vi "Transmit ACK.vi"(8 "error in (no error)":errorcluster, 11 "Client Proxy LNA in":refnum<class "Client Proxy LNA.lvclass">) -> (0 "error out":errorcluster, 3 "Client Proxy LNA out":refnum<class "Client Proxy LNA.lvclass">)   [LabVIEW 2026, in "Client Proxy LNA.lvlib" / "Client Proxy LNA.lvclass"]
uses:
  Client Proxy LNA.lvclass
  C:/Users/E2013170/Documents/GitHub/Measurement-Utility-Reference/recovery/packages/ni_lib_linked_network_actor-1.2.0.19-9492AF5A82/File Group 0/vi.lib/NI/Actors/Linked Network Actor/Linked Network Actor/Linked Network Actor.lvclass
  Client Proxy LNA.lvclass/Client Proxy LNA.ctl
  recovery/packages/ni_lib_linked_network_actor-1.2.0.19-9492AF5A82/File Group 0/vi.lib/NI/Actors/Linked Network Actor/Linked Network Actor/Linked Network Actor.lvclass/Linked Network Actor.ctl
  recovery/packages/ni_lib_linked_network_actor-1.2.0.19-9492AF5A82/File Group 0/vi.lib/NI/Actors/Linked Network Actor/Linked Network Actor/Linked Network Actor.lvclass
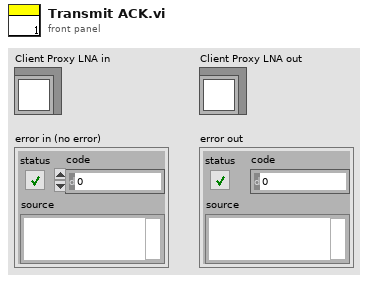
[diagram p1: front panel]
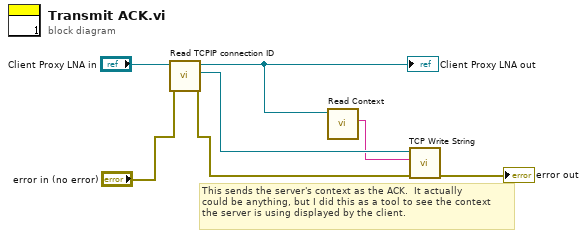
[diagram p0: block diagram]
diagram:
  # "This sends the server's context as the ACK.  It actually\ncould be anything, but I did this as a tool to see the context\nthe server is using displayed by the client."
  n1 = call "Read TCPIP connection ID.vi"("error in (no error)"="error in (no error)", "Client Proxy LNA in"="Client Proxy LNA in") -> ("error out"=w6:errorcluster, "TCPIP connection ID"=w3:refnum<k5>, "Client Proxy LNA out"=w1:refnum<class "Client Proxy LNA.lvclass">)  [unwired: 7 in]
  "Client Proxy LNA out" <- w1
  n2 = call "Read Context.vi"("Linked Network Actor in"=w1) -> ("Context"=w2:string)  [unwired: 10 in]
  n3 = call "TCP Write String.vi"("error in (no error)"=w6, "data in"=w2, "connection ID"=w3) -> ("error out"=→"error out":errorcluster)  [unwired: 7 in, 1 out]
